vi "Default Settings.vi"(6 "Assembly Type":string, 8 "error in (no error)":errorcluster, 11 "Sensor Dispense in":refnum<class "Sensor Dispense.lvclass">) -> (0 "error out":errorcluster, 3 "Sensor Dispense out":refnum<class "Sensor Dispense.lvclass">)   [LabVIEW 2021, in "Sensor Dispense.lvclass"]
uses:
  Projects/Sensor Dispense.lvclass
  C:/Users/HEP/Documents/GitHub/Gantry/UCSB-Gantry-HEP-main/Classes/Routine/Dispense/Dispense.lvclass
  Projects/Sensor Dispense.lvclass/Sensor Dispense.ctl
  Dispense.lvclass/Dispense.ctl
  Write Tip Height.vi
  <vilib>/Utility/file.llb/Read Delimited Spreadsheet (string).vi
  Dispense.lvclass
panel:
  in  "Dispense Type":u16
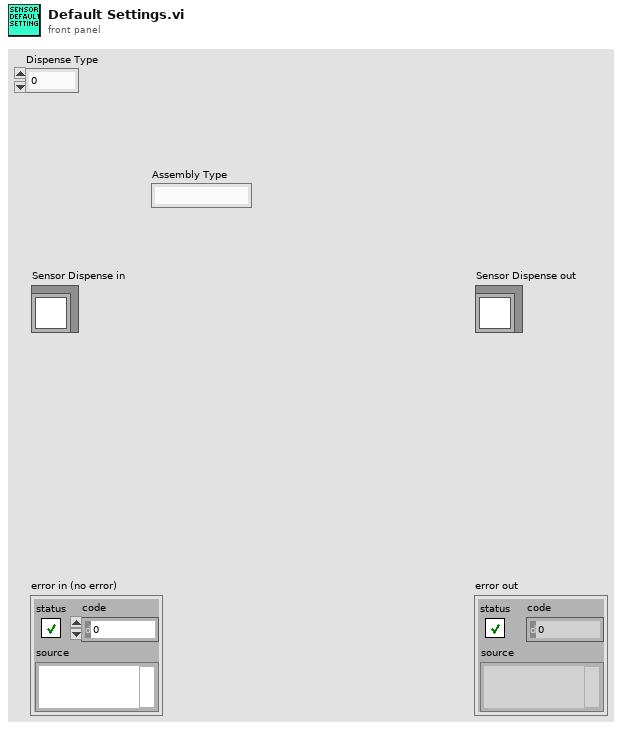
[diagram p1: front panel]
types:
  T1 = typedef "File Paths.ctl" = cluster{"Glue Pattern Folder":path, "Carrier Tray Folder":path, "Pick Up Tool Fixture Folder":path, "Components Folder":path, "Bellows Tool Offset.txt":path, "Pick Up Tool Offset.txt":path, "Dispense Tip Offset.txt":path, "Log Files":path, "Gantry Assembly Map.txt":path, "Syringe and offset map.txt":path, "Controllers Folder":path, "Local dbase config":path}
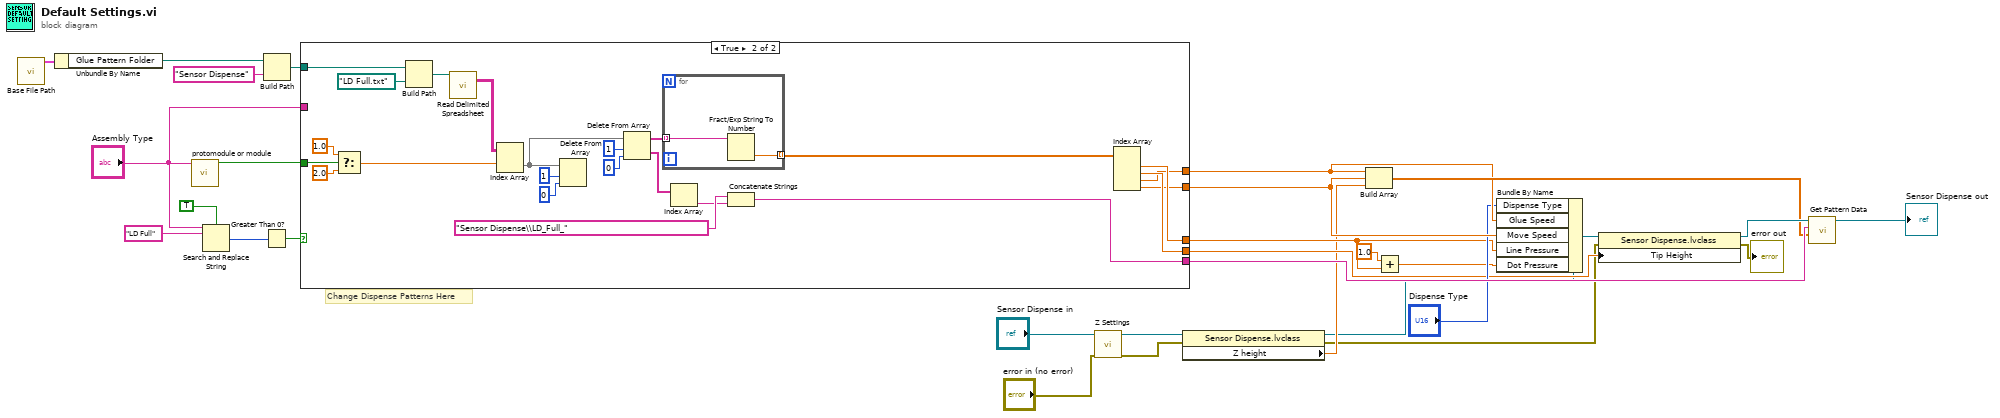
[diagram p0: block diagram]
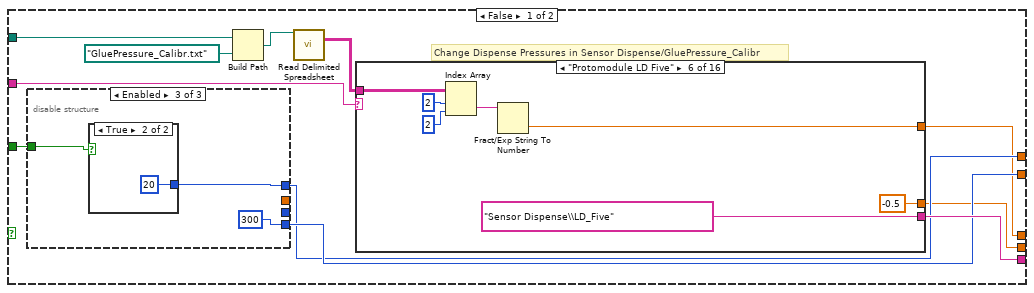
[diagram p2: hidden frame]
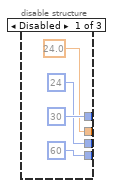
[diagram p3: hidden frame]
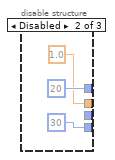
[diagram p4: hidden frame]
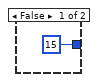
[diagram p5: hidden frame]
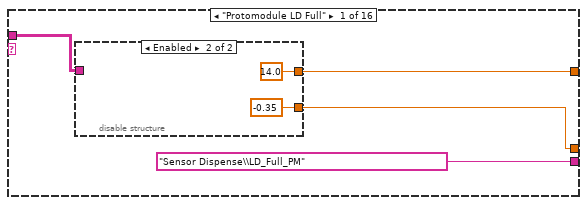
[diagram p6: hidden frame]
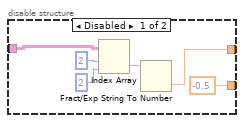
[diagram p7: hidden frame]
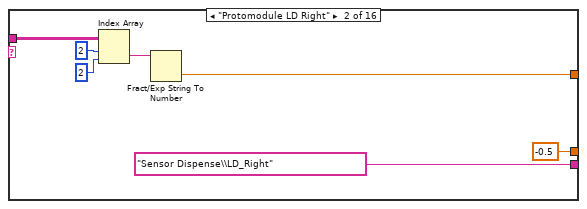
[diagram p8: hidden frame]
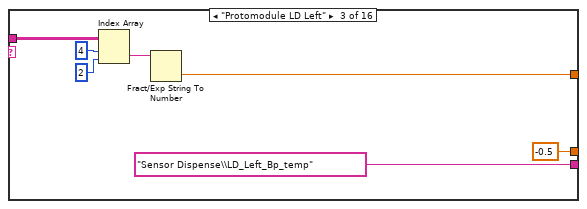
[diagram p9: hidden frame]
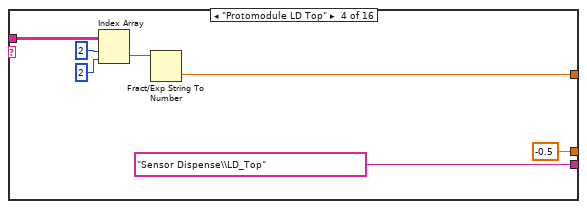
[diagram p10: hidden frame]
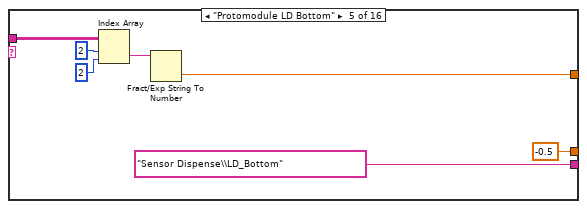
[diagram p11: hidden frame]
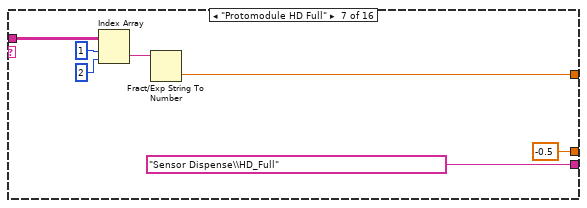
[diagram p12: hidden frame]
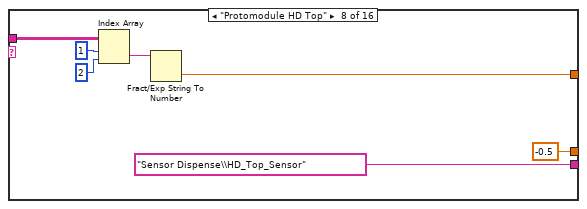
[diagram p13: hidden frame]
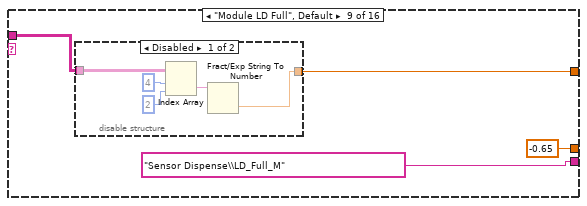
[diagram p14: hidden frame]
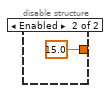
[diagram p15: hidden frame]
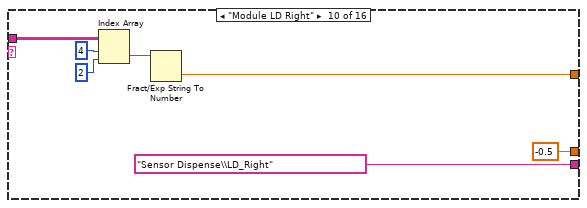
[diagram p16: hidden frame]
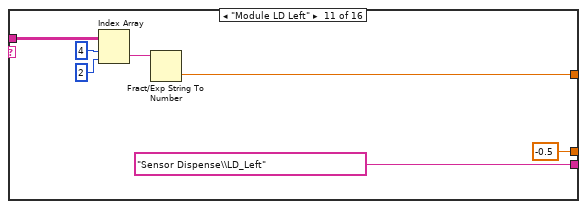
[diagram p17: hidden frame]
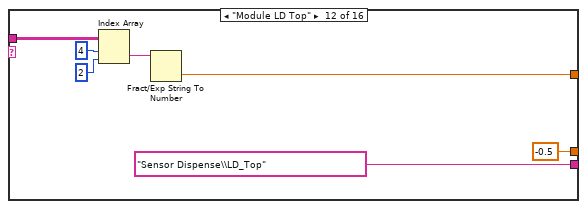
[diagram p18: hidden frame]
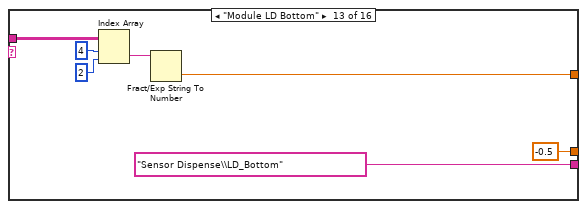
[diagram p19: hidden frame]
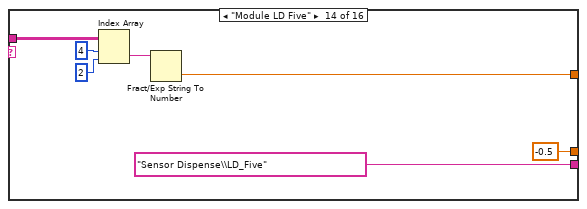
[diagram p20: hidden frame]
diagram:
  # "Change Dispense Patterns Here"
  n1 = call "Base File Path.vi"() -> ("Paths Out"=w19:T1)  [unwired: 11 in]
  n2 = Unbundle By Name(w19) -> ("Glue Pattern Folder"=w18:path)
  n3 = call "protomodule or module.vi"("assembly type"="Assembly Type") -> ("protomodule? (T)"=w2:bool)  [unwired: 10 in]
  n4 = Search and Replace String(case sensitive?=TRUE ("ignore case? (F)"), input string="Assembly Type", search string="LD Full") -> (number of replacements=w8:i32)  [unwired: 5 in, 3 out]
  n5 = Greater Than 0?(x=w8) -> (x > 0?=w4:bool)
  n6 = Build Path(base path=w18, name or relative path="Sensor Dispense") -> (appended path=w3:path)
  n7 = case shown="True" w4 {
    tunnel: [w41 w185] -> w28
    tunnel: [w40 w174] -> w24
    tunnel: [w39 w175] -> w23
    tunnel: [w38 w177] -> w20
    tunnel: [w37 w176] -> w16
    tunnel: "Assembly Type" -> [w36 _]
    tunnel: w3 -> [w33 w196]
    tunnel: w2 -> [w31 w192]
    frame False {
      # "Change Dispense Pressures in Sensor Dispense/GluePressure_Calibr"
      n8 = disable-structure shown="Enabled" {
        disable-tunnel: [60 30 300] -> w40
        disable-tunnel: [30 20 w50] -> w39
        disable-tunnel: [24.0 ("Dot Pressure") 1.0 ("Dot Pressure") _] -> _
        disable-tunnel: [24 _ _] -> _
        disable-tunnel: w31 -> [_ _ w49]
        frame Disabled {
        }
        frame Disabled {
        }
        frame Enabled {
          n9 = case shown="True" w49 {
            tunnel: [15 20] -> w50
            frame False {
            }
            frame True {
            }
          }
        }
      }
      n10 = Build Path(base path=w33, name or relative path=path "GluePressure_Calibr.txt") -> (appended path=w35:path)
      n11 = call-poly <vilib>:"Read Delimited Spreadsheet.vi"("file path (dialog if empty)"=w35) -> ("all rows"=w32:string[][])  [unwired: 9 in, 5 out]
      n12 = case shown="\"Protomodule LD Five\"" w36 {
        tunnel: ["Sensor Dispense\\LD_Full_PM" "Sensor Dispense\\LD_Right" "Sensor Dispense\\LD_Left_Bp_temp" "Sensor Dispense\\LD_Top" "Sensor Dispense\\LD_Bottom" "Sensor Dispense\\LD_Five" "Sensor Dispense\\HD_Full" "Sensor Dispense\\HD_Top_Sensor" "Sensor Dispense\\LD_Full_M" "Sensor Dispense\\LD_Right" "Sensor Dispense\\LD_Left" "Sensor Dispense\\LD_Top" "Sensor Dispense\\LD_Bottom" "Sensor Dispense\\LD_Five" "Sensor Dispense\\HD_Top_HB" "Sensor Dispense\\HD_Full"] -> w41
        tunnel: [w55 w67 w74 w81 w88 w95 w102 w109 w116 w126 w133 w140 w147 w154 w161 w168] -> w38
        tunnel: w32 -> [w56 w68 w75 w82 w89 w96 w103 w110 w117 w127 w137 w141 w148 w155 w162 w169]
        tunnel: [w54 -0.5 -0.5 -0.5 -0.5 -0.5 -0.5 -0.5 -0.65 -0.5 -0.5 -0.5 -0.5 -0.5 -0.5 -0.5] -> w37
        frame "Protomodule LD Full" {
          n13 = disable-structure shown="Enabled" {
            disable-tunnel: w56 -> [w60 _]
            disable-tunnel: [w59 14.0] -> w55
            disable-tunnel: [-0.5 -0.35] -> w54
            frame Disabled {
              n14 = Index Array(array=w60, index (row)=2, index (col)=2 ("index (row)")) -> (element=w61:string)
              n15 = Fract/Exp String To Number(string=w61) -> (number=w59:dbl)  [unwired: 3 in, 1 out]
            }
            frame Enabled {
            }
          }
        }
        frame "Protomodule LD Right" {
          n16 = Index Array(array=w68, index (row)=2, index (col)=2 ("index (row)")) -> (element=w71:string)
          n17 = Fract/Exp String To Number(string=w71) -> (number=w67:dbl)  [unwired: 3 in, 1 out]
        }
        frame "Protomodule LD Left" {
          n18 = Index Array(array=w75, index (row)=4, index (col)=2 ("index (row)")) -> (element=w76:string)
          n19 = Fract/Exp String To Number(string=w76) -> (number=w74:dbl)  [unwired: 3 in, 1 out]
        }
        frame "Protomodule LD Top" {
          n20 = Index Array(array=w82, index (row)=2, index (col)=2 ("index (row)")) -> (element=w83:string)
          n21 = Fract/Exp String To Number(string=w83) -> (number=w81:dbl)  [unwired: 3 in, 1 out]
        }
        frame "Protomodule LD Bottom" {
          n22 = Index Array(array=w89, index (row)=2, index (col)=2 ("index (row)")) -> (element=w90:string)
          n23 = Fract/Exp String To Number(string=w90) -> (number=w88:dbl)  [unwired: 3 in, 1 out]
        }
        frame "Protomodule LD Five" {
          n24 = Index Array(array=w96, index (row)=2, index (col)=2 ("index (row)")) -> (element=w97:string)
          n25 = Fract/Exp String To Number(string=w97) -> (number=w95:dbl)  [unwired: 3 in, 1 out]
        }
        frame "Protomodule HD Full" {
          n26 = Index Array(array=w103, index (row)=1, index (col)=2 ("index (row)")) -> (element=w104:string)
          n27 = Fract/Exp String To Number(string=w104) -> (number=w102:dbl)  [unwired: 3 in, 1 out]
        }
        frame "Protomodule HD Top" {
          n28 = Index Array(array=w110, index (row)=1, index (col)=2 ("index (row)")) -> (element=w111:string)
          n29 = Fract/Exp String To Number(string=w111) -> (number=w109:dbl)  [unwired: 3 in, 1 out]
        }
        frame "Module LD Full", Default {
          n30 = disable-structure shown="Disabled" {
            disable-tunnel: w117 -> [w120 _]
            disable-tunnel: [w119 15.0] -> w116
            frame Disabled {
              n31 = Index Array(array=w120, index (row)=4, index (col)=2 ("index (row)")) -> (element=w121:string)
              n32 = Fract/Exp String To Number(string=w121) -> (number=w119:dbl)  [unwired: 3 in, 1 out]
            }
            frame Enabled {
            }
          }
        }
        frame "Module LD Right" {
          n33 = Index Array(array=w127, index (row)=4, index (col)=2 ("index (row)")) -> (element=w128:string)
          n34 = Fract/Exp String To Number(string=w128) -> (number=w126:dbl)  [unwired: 3 in, 1 out]
        }
        frame "Module LD Left" {
          n35 = Index Array(array=w137, index (row)=4, index (col)=2 ("index (row)")) -> (element=w134:string)
          n36 = Fract/Exp String To Number(string=w134) -> (number=w133:dbl)  [unwired: 3 in, 1 out]
        }
        frame "Module LD Top" {
          n37 = Index Array(array=w141, index (row)=4, index (col)=2 ("index (row)")) -> (element=w142:string)
          n38 = Fract/Exp String To Number(string=w142) -> (number=w140:dbl)  [unwired: 3 in, 1 out]
        }
        frame "Module LD Bottom" {
          n39 = Index Array(array=w148, index (row)=4, index (col)=2 ("index (row)")) -> (element=w149:string)
          n40 = Fract/Exp String To Number(string=w149) -> (number=w147:dbl)  [unwired: 3 in, 1 out]
        }
        frame "Module LD Five" {
          n41 = Index Array(array=w155, index (row)=4, index (col)=2 ("index (row)")) -> (element=w156:string)
          n42 = Fract/Exp String To Number(string=w156) -> (number=w154:dbl)  [unwired: 3 in, 1 out]
        }
        frame "Module HD Top" {
          n43 = Index Array(array=w162, index (row)=3, index (col)=2 ("index (row)")) -> (element=w165:string)
          n44 = Fract/Exp String To Number(string=w165) -> (number=w161:dbl)  [unwired: 3 in, 1 out]
        }
        frame "Module HD Full" {
          n45 = Index Array(array=w169, index (row)=3, index (col)=2 ("index (row)")) -> (element=w170:string)
          n46 = Fract/Exp String To Number(string=w170) -> (number=w168:dbl)  [unwired: 3 in, 1 out]
        }
      }
    }
    frame True {
      n47 = Select(t=1.0, s=w192, f=2.0) -> (s? t:f=w191:dbl)
      n48 = Build Path(base path=w196, name or relative path=path "LD Full.txt") -> (appended path=w194:path)
      n49 = call-poly <vilib>:"Read Delimited Spreadsheet.vi"("file path (dialog if empty)"=w194) -> ("all rows"=w193:string[][])  [unwired: 9 in, 5 out]
      n50 = Index Array(array=w193, index (row)=w191) -> (element=w184:string[])  [unwired: 1 in]
      n51 = Delete From Array(array=w184, length=1, index=0) -> ()  [unwired: 2 out]
      n52 = Delete From Array(array=w184, length=1, index=0) -> (deleted portion=w181:string[], array with subset deleted=w179:string[])
      n53 = for {
        tunnel: w179 -> [w198] mode=indexing
        tunnel: [w197] -> w178 mode=indexing
        n54 = Fract/Exp String To Number(string=w198) -> (number=w197:dbl)  [unwired: 3 in, 1 out]
      }
      n55 = Index Array(array=w181) -> (element=w180:string)  [unwired: 1 in]
      n56 = Concatenate Strings("Sensor Dispense\\LD_Full_", w180) -> (w185:string)
      n57 = Index Array(array=w178) -> (element #1=w177:dbl, element #2=w176:dbl, element #3=w175:dbl, element #4=w174:dbl)  [unwired: 4 in]
    }
  }
  n58 = call-dynamic "Z Settings.vi"("error in (no error)"="error in (no error)", "Dispense in"="Sensor Dispense in") -> ("error out"=w11:errorcluster, "Dispense out"=w9:refnum<class "Sensor Dispense.lvclass">)  [unwired: 8 in]
  n59 = property class="Sensor Dispense.lvclass"(reference=w9, error in=w11) -> (reference out=w14:refnum<class "Sensor Dispense.lvclass">, error out=w13:errorcluster, "Z height"=w15:dbl)
  n60 = Build Array(w23, w24, w15) -> (w27:dbl[])
  n61 = Add(x=1.0 ("Dot Pressure"), y=w20) -> (x+y=w21:dbl)
  n62 = Bundle By Name(cluster=w14, "Dispense Type"="Dispense Type", "Glue Speed"=w23, "Move Speed"=w24, "Line Pressure"=w20, "Dot Pressure"=w21) -> (w30:refnum<class "Sensor Dispense.lvclass">)
  n63 = property class="Sensor Dispense.lvclass"(reference=w30, error in=w13, "Tip Height"=w16) -> (reference out=w29:refnum<class "Sensor Dispense.lvclass">, error out=→"error out":errorcluster)
  n64 = call "Get Pattern Data.vi"("File Name"=w27, "Folder Name"=w28, "Dispense.lvclass"=w29) -> ("Dispense Out"=→"Sensor Dispense out":refnum<class "Sensor Dispense.lvclass">)  [unwired: 8 in]
